vi "Close PJVS.vi"(8 "error in (pass through)":errorcluster, 11 "PJVS setup":T1={"PJVS type"=enum."AC-supraVOLTcontrol", "Status Refnum"=refnum, "Abort Refnum"=refnum, "AC-supraVOLTcontrol"={"IP address:port (0.0.0.0:0000)"="0.0.0.0:0000", "Timeouts"={"TCP Read & Write (ms)"=7000, "Sensors readout"=5000, "PJVS setup"=10000, "Nullmeter readout"=5000, "Multiplexer setup"=3000, "57XX setup"=15000, "Generator setup"=5000, "Synthesizer setup"=3000, "Sampler readout"=10000}, "Simulation mode"=FALSE, "Debug mode"=FALSE}, "NPL bias source"={"DataSocketCluster"={"Server Machine"="CZC", "Client Machine"="localhost", "Data"="P2", "TimeStamp"=0.0, "Count"=1, "Target Process"="General Server"}}} {"NPL bias source"."DataSocketCluster"."TimeStamp" format="%.2f"}) -> (0 "error out":errorcluster, 3 "PJVS setup out":T1={"PJVS type"=enum."AC-supraVOLTcontrol", "Status Refnum"=refnum, "Abort Refnum"=refnum, "AC-supraVOLTcontrol"={"IP address:port (0.0.0.0:0000)"="0.0.0.0:0000", "Timeouts"={"TCP Read & Write (ms)"=7000, "Sensors readout"=5000, "PJVS setup"=10000, "Nullmeter readout"=5000, "Multiplexer setup"=3000, "57XX setup"=15000, "Generator setup"=5000, "Synthesizer setup"=3000, "Sampler readout"=10000}, "Simulation mode"=FALSE, "Debug mode"=FALSE}, "NPL bias source"={"DataSocketCluster"={"Server Machine"="CZC", "Client Machine"="localhost", "Data"="P2", "TimeStamp"=0.0, "Count"=1, "Target Process"="General Server"}}} {"NPL bias source"."DataSocketCluster"."TimeStamp" format="%.2f"})   [LabVIEW 2020]
doc: "Initialize the PJVS. Calls the initialization routine of the actual driver."
uses:
  Type definitions/PJVS Type.ctl
  Type definitions/PJVS Setup.ctl
  PJVS drivers/acsvcontrol-driver/build/ACSVcontrol-driver_0.2.0.0.llb/Timeouts.ctl
  PJVS drivers/acsvcontrol-driver/build/ACSVcontrol-driver_0.2.0.0.llb/ACSVcontrol-driver.lvlib
  PJVS drivers/JV modified NPL Bias source/DataSocketCluster external.ctl
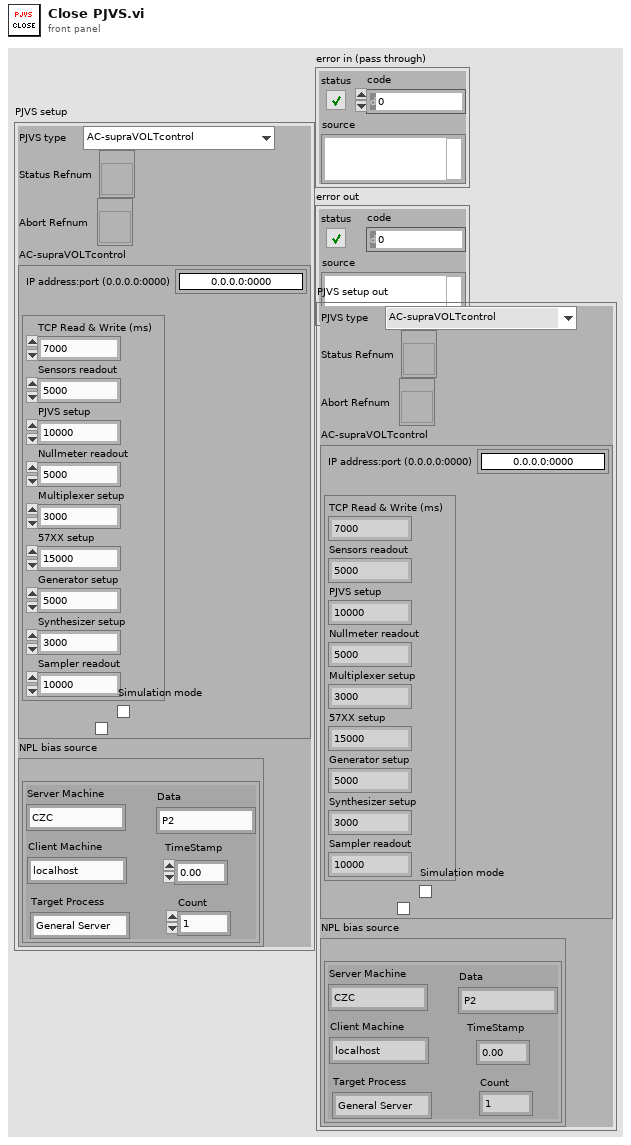
[diagram p1: front panel]
types:
  T1 = typedef "PJVS Setup.ctl" = cluster{"PJVS type":T2, "Status Refnum":refnum<vi>, "Abort Refnum":refnum<vi>, "AC-supraVOLTcontrol":cluster{"IP address:port (0.0.0.0:0000)":string, "Timeouts":T3, "Simulation mode":bool, "Debug mode":bool}, "NPL bias source":cluster{"DataSocketCluster":T4}}
  T2 = typedef "PJVS Type.ctl" = enum16{"AC-supraVOLTcontrol", "JV modified NPL bias control"}
  T3 = typedef "ACSVcontrol-driver.lvlib/Timeouts.ctl" = cluster{"TCP Read & Write (ms)":i32, "Sensors readout":i32, "PJVS setup":i32, "Nullmeter readout":i32, "Multiplexer setup":i32, "57XX setup":i32, "Generator setup":i32, "Synthesizer setup":i32, "Sampler readout":i32}
  T4 = typedef "DataSocketCluster external.ctl" = cluster{"Server Machine":string, "Client Machine":string, "Data":string, "TimeStamp":dbl, "Count":i32, "Target Process":string}
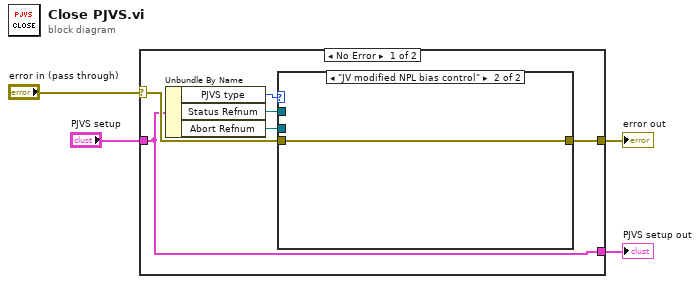
[diagram p0: block diagram]
diagram:
  n1 = case shown="No Error" "error in (pass through)" {
    selector: "error in (pass through)" -> [w6 w14]
    tunnel: "PJVS setup" -> [w5 w13]
    tunnel: [w7 w14] -> w3
    tunnel: [w5 w13] -> w1
    frame No Error {
      n2 = Unbundle By Name(w5) -> ("PJVS type"=w10:T2, "Status Refnum"=w9:refnum<vi>, "Abort Refnum"=w8:refnum<vi>)
      n3 = case shown="\"JV modified NPL bias control\"" w10 {
        tunnel: w9 -> [_ _]
        tunnel: w8 -> [_ _]
        tunnel: w6 -> [w11 w12]
        tunnel: [w11 w12] -> w7
        frame "AC-supraVOLTcontrol", Default {
        }
        frame "JV modified NPL bias control" {
        }
      }
    }
    frame Error {
    }
  }
  "error out" <- w3
  "PJVS setup out" <- w1
